vi "CSM - List Rules in Broadcast Registry.vi"(8 "error in (no error)":errorcluster) -> (0 "error out":errorcluster, 2 "Rule Entries with Register Type":T2(array[cluster]), 3 "Rule Entries":T3(array[cluster]))   [LabVIEW 2017, in "Communicable State Machine.lvlib"]
doc: "Lists all rules in the CSM registry.\n\n\n> [!NOTE] <b>CSM Broadcast</b>\n>\n> Broadcasts in CSM are divided into three types: Status Broadcast, Interrupt Broadcast, and State Broadcast. The module pushes the Status Broadcast to all modules registered to that Status Broadcast. Status Broadcast and Interrupt Broadcast are explicitly called broadcasts, while State Broadcast is an implicit broadcast. When a registration relationship exists, the State Broadcast is automatically triggered when the CSM completes a certain state.\n> - <b>Status Broadcast</b>: Normal priority broadcast. Similar to asynchronous messages, it is passed via the low-priority queue. It is processed sequentially when other unprocessed asynchronous messages or Status Broadcasts exist in the module.\n> - <b>Interrupt Broadcast</b>: High priority broadcast. Similar to synchronous messages, it is passed via the high-priority queue. It is processed first when other low-priority asynchronous messages or Status Broadcasts exist in the module. However, if other unprocessed synchronous messages or Interrupt Broadcasts exist, it is processed sequentially.\n> - <b>State Broadcast</b>: State Broadcast is an implicit broadcast. When a registration relationship exists, the State Broadcast is automatically triggered when the CSM completes a certain state. The argument for the State Broadcast is the Response of the CSM state.\n> <b>Note</b>:\n> - Status broadcasts or interrupt broadcasts must be explicitly sent. Do not use names identical to CSM state names. Otherwise, multiple triggers may occur.\n> - For efficiency considerations, state broadcasts are only sent when registered to. This means you must register to receive state broadcasts in a module's broadcast events.\n\n\n> [!NOTE] <b>CSM Registration</b>\n>\n> Registration associates a broadcast with a bound interface (API). When the broadcast is triggered, the bound interface (API) is called. Registrations can also be cancelled. In CSM, there are two types of broadcasts:\n>\n> - <b>Broadcast</b>: Broadcast explicitly called by the module sending the broadcast message. Arguments need to be explicitly provided.\n> - <b>State</b>: Any state of a CSM module can also be registered to. The argument received by the triggered API is the Response of the CSM state.\n>\n> // Register\n> [CSM Broadcast]@[SourceModule] >> [Bound API]@[TargetModule] -><register> // [Comments]\n> // Unregister\n> [CSM Broadcast]@[SourceModule] >> [Bound API]@[TargetModule] -><unregister> // [Comments]\n>\n> - <b>CSM Broadcast</b>: Defined by the source module. Refer to \"CSM Broadcast Format Parsing\" for details.\n> - <b>Source Module</b>: The broadcasting module. If registering to broadcasts from any module, the source module can be represented by `*`.\n> - <b>Bound API</b>: Defined by the target module. It is the external interface of the target module.\n> - <b>Target Module</b>: The module where the bound API resides. When indicating registration to the current module within a CSM module, it can be ignored. The preceding `@` separator is also omitted.\n> - `<register>` / `<unregister>`: Definition of the Register/Unregister operation type.\n> - <b>Comments</b>: Comment information, which will not be parsed.\n\n\n-- <b>Indicators</b> --\n- <b>Rule Entries</b>: All rule entries."
uses:
  Communicable State Machine.lvlib
  CSM - Broadcast Message Type.ctl
  _Support/FGV-BroadcastRegistry/Operation-BroadcastRegistry.ctl
  _Shared/CSM Shared.lvlib
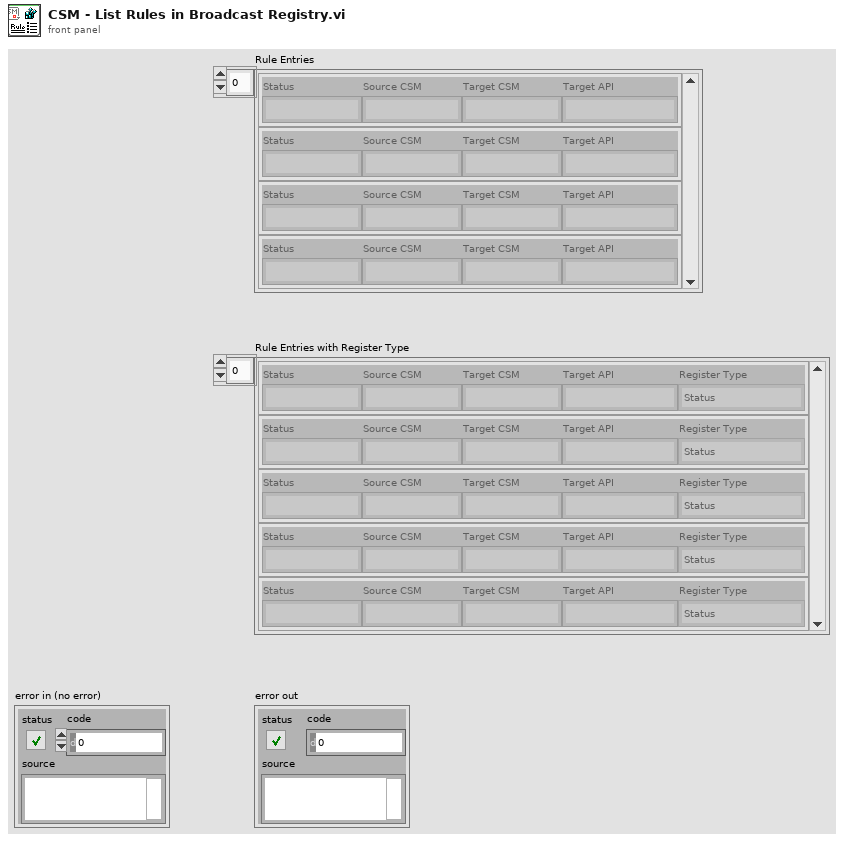
[diagram p1: front panel]
types:
  T1 = typedef "Communicable State Machine.lvlib/CSM - Broadcast Message Type.ctl" = enum16{"<Null>", "Status", "Interrupt"}
  T2 = cluster{"Status":string, "Source CSM":string, "Target CSM":string, "Target API":string, "Register Type":T1}[]
  T3 = cluster{"Status":string, "Source CSM":string, "Target CSM":string, "Target API":string}[]
  T4 = typedef "Communicable State Machine.lvlib/Operation-BroadcastRegistry.ctl" = enum16{"Delete Source Module", "Delete Target Module", "Remove Module", "Register", "Unregister", "Check", "List Status", "List Entries", "List Status Of Source", "Drop", "Register As Status", "Register As Interrupt"}
  T5 = cluster{"Status":string, "Source CSM":string, "Target CSM":string, "Target API":string, "Register Type":T1}
  T6 = cluster{"Status":string, "Source CSM":string, "Target CSM":string, "Target API":string}
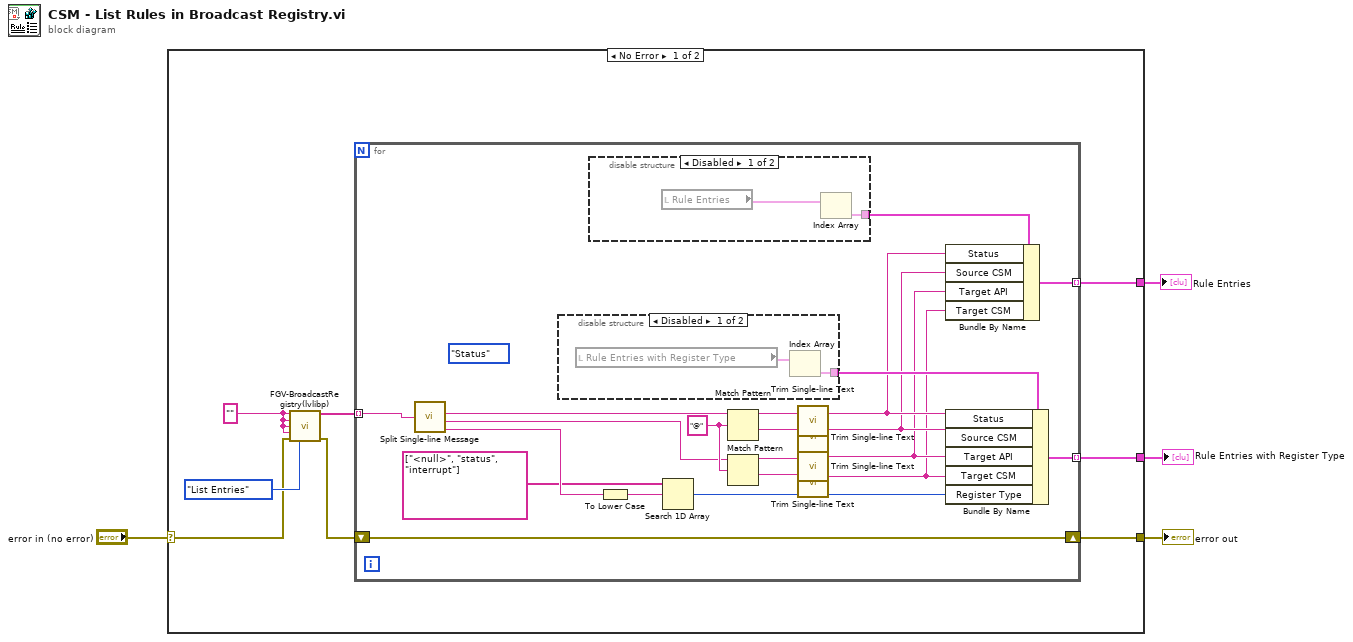
[diagram p0: block diagram]
diagram:
  n1 = case shown="No Error" "error in (no error)" {
    selector: "error in (no error)" -> [w10 w38]
    tunnel: [w12 w38] -> w4
    tunnel: [w7 _] -> w2
    tunnel: [w5 _] -> w1
    frame No Error {
      w8 = "" ("Source")
      n2 = call "FGV-BroadcastRegistry(lvlibp).vi"("Source"=w8, "Target"=w8, "Status"=w8, "API"=w8, "Error In"=w10, "Operation"=Operation-BroadcastRegistry."List Entries") -> ("Response Message"=w6:string[], "error out"=w9:errorcluster)  [unwired: 7 in, 1 out]
      n3 = for {
        shift-right: [w33] -> w12
        shift-left: w9 -> [w33]
        tunnel: [w30] -> w7 mode=indexing
        tunnel: w6 -> [w25] mode=indexing
        tunnel: [w17] -> w5 mode=indexing
        (unwired) CSM_-_Broadcast_Message_Type."Status" ("Register Type")
        w32 = "@" ("regular expression")
        n4 = call "Split Single-line Message.vi"("single-line text"=w25) -> ("state"=w24:string, "args"=w23:string, "source/target"=w22:string)  [unwired: 6 in, 1 out]
        n5 = disable-structure shown="Disabled" {
          disable-tunnel: [w36 _] -> w31
          frame Disabled {
            n6 = local read "Rule Entries with Register Type"() -> (w37:T2)
            n7 = Index Array(array=w37) -> (element=w36:T5)  [unwired: 1 in]
          }
          frame Enabled {
          }
        }
        n8 = disable-structure shown="Disabled" {
          disable-tunnel: [w34 _] -> w18
          frame Disabled {
            n9 = local read "Rule Entries"() -> (w35:T3)
            n10 = Index Array(array=w35) -> (element=w34:T6)  [unwired: 1 in]
          }
          frame Enabled {
          }
        }
        n11 = To Lower Case(string=w22) -> (all lower case string=w19:string)
        n12 = Search 1D Array(1D array=string[] ["<null>", "status", "interrupt"] ("Source"), element=w19) -> (index of element=w21:i32)  [unwired: 1 in]
        n13 = Match Pattern(string=w24, regular expression=w32) -> (before substring=w29:string, after substring=w28:string)  [unwired: 1 in, 2 out]
        n14 = Match Pattern(string=w23, regular expression=w32) -> (before substring=w27:string, after substring=w26:string)  [unwired: 1 in, 2 out]
        n15 = call "Trim Single-line Text.vi"("single-line text"=w29) -> ("trimed text"=w16:string)  [unwired: 2 in]
        n16 = call "Trim Single-line Text.vi"("single-line text"=w28) -> ("trimed text"=w15:string)  [unwired: 2 in]
        n17 = call "Trim Single-line Text.vi"("single-line text"=w27) -> ("trimed text"=w14:string)  [unwired: 2 in]
        n18 = call "Trim Single-line Text.vi"("single-line text"=w26) -> ("trimed text"=w13:string)  [unwired: 2 in]
        n19 = Bundle By Name(cluster=w18, "Status"=w16, "Source CSM"=w15, "Target API"=w14, "Target CSM"=w13) -> (w17:T6)
        n20 = Bundle By Name(cluster=w31, "Status"=w16, "Source CSM"=w15, "Target API"=w14, "Target CSM"=w13, "Register Type"=w21) -> (w30:T5)
      }
    }
    frame Error {
    }
  }
  "Rule Entries" <- w1
  "error out" <- w4
  "Rule Entries with Register Type" <- w2
